vi "ExSubADCSpeeds.vi"(3 "error in (no error)":errorcluster, 5 "Camera handle":u32) -> (0 "error out":errorcluster, 1 "ADC Speeds":dbl[](array[numeric]) format="%.2p", 2 "Camera handle":u32)   [LabVIEW 2010]
doc: "This subVI returns the available ADC speeds in Hertz in an array. The array index corresponds to the index of the Speed Table. If the camera has multiple output ports, the ADC Speeds array may have multiple entries of the same frequency."
panel:
  # "ExSubADCSpeeds.vi: this sub VI sets the ADC speed of the\ncamera."
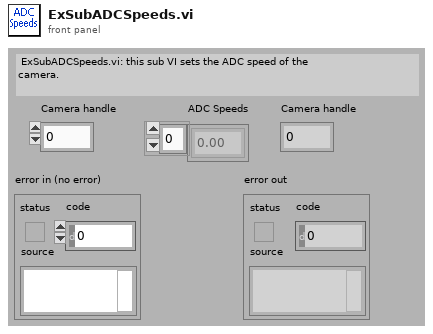
[diagram p1: front panel]
types:
  T1 = cluster{"Param ID":u32, "Avail Flag":u8, "Current Value":dbl, "Default Value":dbl, "Min Value":dbl, "Max Value":dbl, "Increment":dbl, "Data Type":u32, "Access Type":u32, "Bit Used Flag":u32, "Number of Enums":u32, "Description":string}
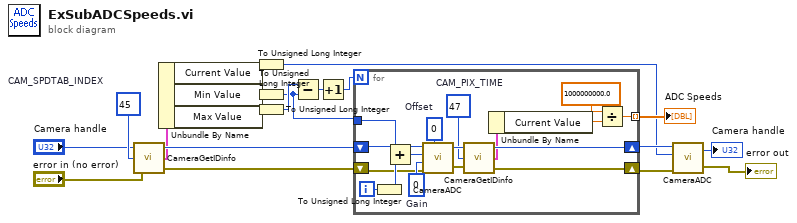
[diagram p0: block diagram]
diagram:
  w18 = u32 45  # CAM_SPDTAB_INDEX
  n1 = call <userlib>:"CameraGetIDinfo.vi"("error in"="error in (no error)", "Param ID"=w18, "Camera handle"="Camera handle") -> ("error out"=w11:errorcluster, "Param ID Information"=w1:T1, "Camera handle"=w12:u32)
  n2 = Unbundle By Name(w1) -> ("Current Value"=w3:dbl, "Min Value"=w17:dbl, "Max Value"=w16:dbl)
  n3 = To Unsigned Long Integer(number=w3) -> (unsigned 32bit integer=w2:u32)
  n4 = To Unsigned Long Integer(number=w17) -> (unsigned 32bit integer=w13:u32)
  n5 = To Unsigned Long Integer(number=w16) -> (unsigned 32bit integer=w15:u32)
  n6 = Subtract(x=w15, y=w13) -> (x-y=w14:u32)
  n7 = Increment(x=w14) -> (x+1=w10:u32)
  n8 = for {
    N: w10 -> [_]
    shift-right: [w36] -> w7
    shift-left: w12 -> [w21]
    shift-right: [w22] -> w6
    shift-left: w11 -> [w20]
    tunnel: [w28] -> w19 mode=indexing
    tunnel: w13 -> [w23]
    i -> [w26]
    w27 = u32 47  # CAM_PIX_TIME
    w34 = u32 0  # Offset
    w35 = u32 0  # Gain
    n9 = To Unsigned Long Integer(number=w26) -> (unsigned 32bit integer=w24:u32)
    n10 = Add(x=w23, y=w24) -> (x+y=w25:u32)
    n11 = call <userlib>:"CameraADC.vi"("Camera Handle"=w21, "Speed"=w25, "Gain"=w35, "error in (no error)"=w20, "Offset"=w34) -> ("Camera Handle"=w32:u32, "error out"=w33:errorcluster)
    n12 = call <userlib>:"CameraGetIDinfo.vi"("error in"=w33, "Param ID"=w27, "Camera handle"=w32) -> ("error out"=w22:errorcluster, "Param ID Information"=w31:T1, "Camera handle"=w36:u32)
    n13 = Unbundle By Name(w31) -> ("Current Value"=w29:dbl)
    n14 = Divide(x=1000000000.0, y=w29) -> (x/y=w28:dbl)
  }
  "ADC Speeds" <- w19
  n15 = call <userlib>:"CameraADC.vi"("Camera Handle"=w7, "Speed"=w2, "error in (no error)"=w6) -> ("Camera Handle"=→"Camera handle":u32, "error out"=→"error out":errorcluster)  [unwired: 2 in]
